vi "vlq-encoder.vi"(5 "x":i32=-128 format="%.0x") -> (2 "Encoded Hex":u32 format="%.0x")   [LabVIEW 2019]
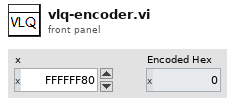
[diagram p1: front panel]
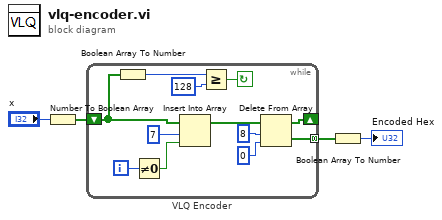
[diagram p0: block diagram]
diagram:
  n1 = Number To Boolean Array(number="x") -> (Boolean array=w2:bool[])
  n2 = while "VLQ Encoder" {
    shift-right: [w6] -> _
    shift-left: w2 -> [w5]
    tunnel: [w7] -> w3 mode=concatenating
    i -> [w13]
    stop <- w8 continue-if-true
    n3 = Boolean Array To Number(Boolean array=w5) -> (number=w10:u32)
    n4 = Not Equal To 0?(x=w13) -> (x != 0?=w12:bool)
    n5 = Insert Into Array(array=w5, index=7, new element=w12) -> (w11:bool[])
    n6 = Greater Or Equal?(x=w10, y=u32 128) -> (x >= y?=w8:bool)
    n7 = Delete From Array(array=w11, length=8, index=0) -> (deleted portion=w7:bool[], array with subset deleted=w6:bool[])
  }
  n8 = Boolean Array To Number(Boolean array=w3) -> (number=→"Encoded Hex":u32)
